vi "센서 라인트레이닝.vi"() -> ()   [LabVIEW 2010]
uses:
  <vilib>/NXT/Subs/MotorOutput.ctl
  <vilib>/NXT/Block Support/NXT_InputPort.ctl
  <vilib>/NXT/Dual Mode Library/Motors/MotorOn.vi
panel:
  in  "빛 센서 포트":T1=2 items=["Port 1", "Port 2", "Port 3", "Port 4"]
  in  "Power (75)":i32=75
  in  "Motor C":T2=3 items=["Port A", "Port B", "Port C", "All Ports"]
  in  "Motor A":T2=3 items=["Port A", "Port B", "Port C", "All Ports"]
  in  "stop":bool
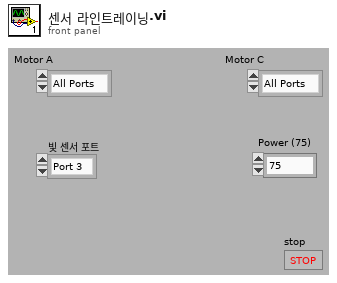
[diagram p1: front panel]
types:
  T1 = typedef "NXT_InputPort.ctl" = u8
  T2 = typedef "MotorOutput.ctl" = u8
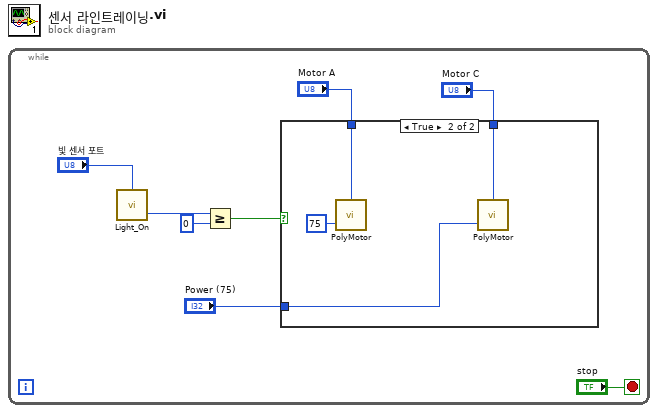
[diagram p0: block diagram]
diagram:
  n1 = while {
    stop <- "stop" stop-if-true
    n2 = call <vilib>:"Light_On.vi"("Port (Port 3)"="빛 센서 포트") -> ("Scaled Value"=w3:i16)  [unwired: 2 in, 1 out]
    n3 = Greater Or Equal?(x=w3, y=i16 0) -> (x >= y?=w4:bool)
    n4 = case shown="True" w4 {
      tunnel: "Motor A" -> [_ w12]
      tunnel: "Motor C" -> [_ w11]
      tunnel: "Power (75)" -> [_ w10]
      frame False {
      }
      frame True {
        n5 = call-poly <vilib>:"PolyMotor.vi"("Power (75)"=75, "Output Port (All Ports)"=w12) -> ()  [unwired: 2 in, 1 out]
        n6 = call-poly <vilib>:"PolyMotor.vi"("Power (75)"=w10, "Output Port (All Ports)"=w11) -> ()  [unwired: 2 in, 1 out]
      }
    }
  }
